vi "值已改变DEMO.vi"() -> ()   [LabVIEW 2012]
panel:
  in  "停止":bool
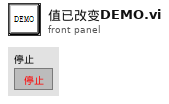
[diagram p1: front panel]
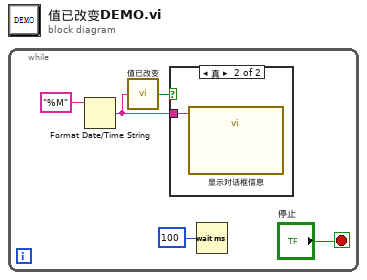
[diagram p0: block diagram]
diagram:
  n1 = while {
    stop <- "停止" stop-if-true
    n2 = Format Date/Time String(time format string (%c)="%M" ("时间格式字符串(%c)")) -> (date/time string=w1:string)  [unwired: 2 in]
    n3 = call-poly "值已改变.vi"("输入数据"=w1) -> ("已更改"=w3:bool)  [unwired: 3 in]
    n4 = case shown="真" w3 {
      tunnel: w1 -> [_ w6]
      frame False {
      }
      frame True {
        n5 = call "显示对话框信息"("Message"=w6) -> ()  [unwired: 9 in, 2 out]
      }
    }
    n6 = Wait (ms)(milliseconds to wait=u32 100 ("等待时间（毫秒）")) -> ()  [unwired: 1 out]
  }
